vi "S-Curve2.vi"(8 "Conditions":T1, 9 "dt (s)":dbl=1.0, 10 "goal":dbl, 11 "Limits":T2) -> (0 "X":dbl[](array[numeric]), 1 "T":dbl[](array[numeric]), 3 "V":dbl[](array[numeric]))   [LabVIEW 2020]
uses:
  sub-vi/Sigmoid.vi
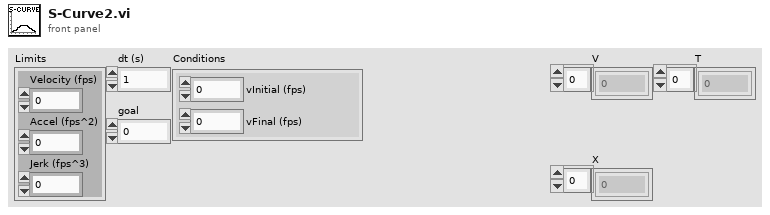
[diagram p1: front panel]
types:
  T1 = cluster{"vInitial (fps)":dbl, "vFinal (fps)":dbl}
  T2 = cluster{"Velocity (fps)":dbl, "Accel (fps^2)":dbl, "Jerk (fps^3)":dbl}
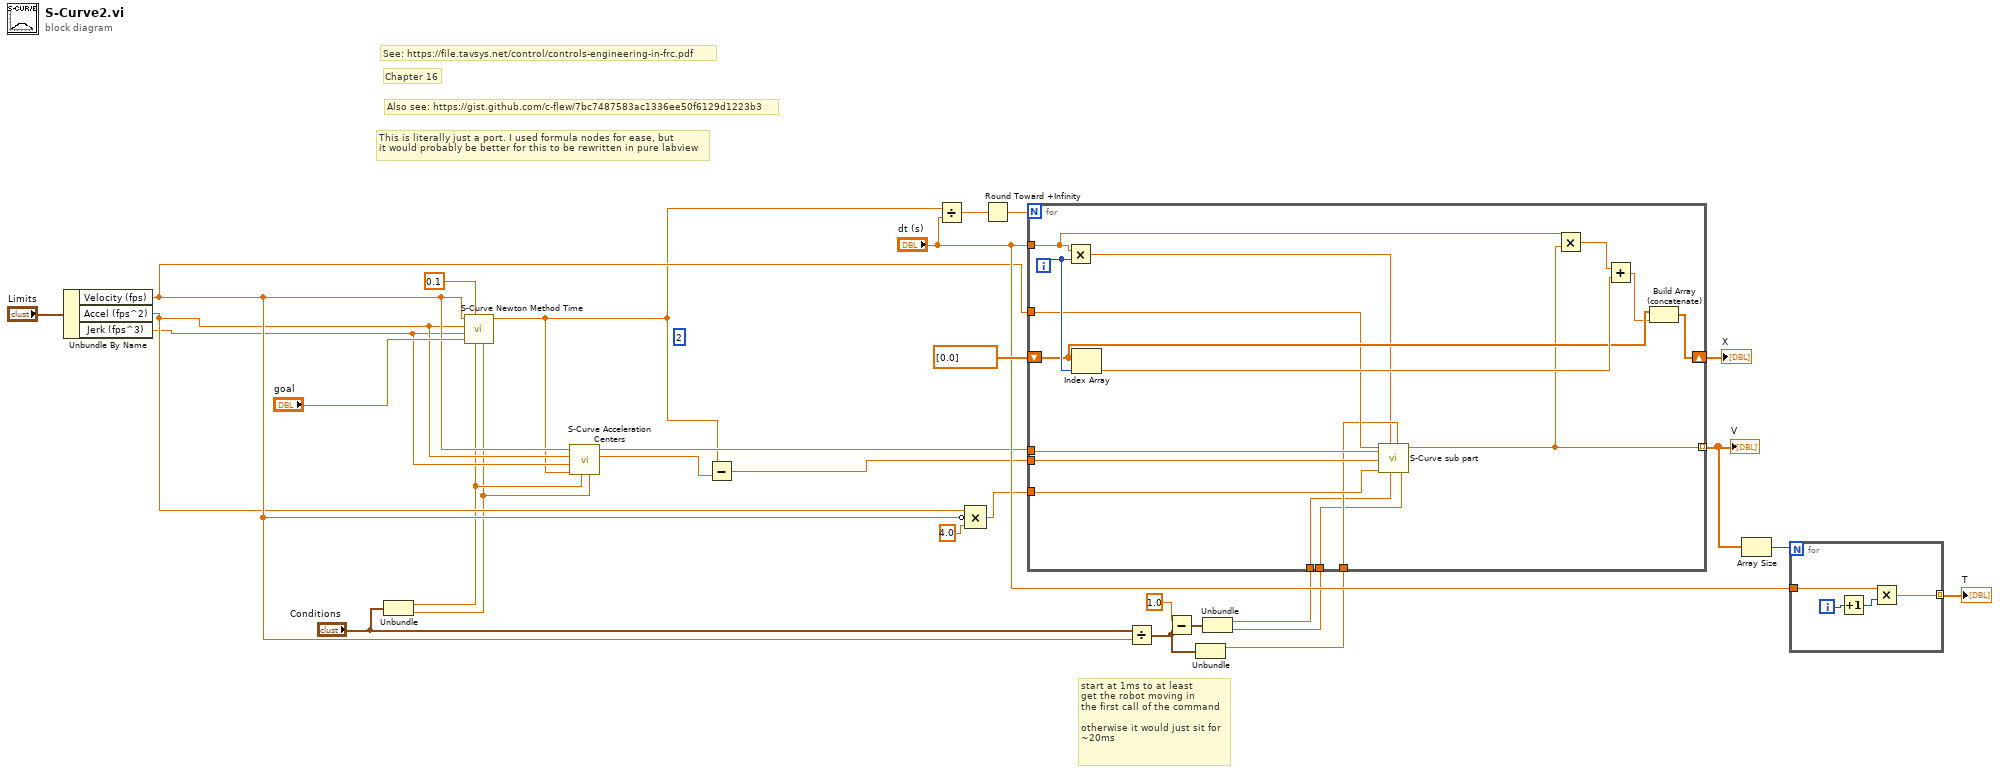
[diagram p0: block diagram]
diagram:
  (unwired) 2
  # "This is literally just a port. I used formula nodes for ease, but\nit would probably be better for this to be rewritten in pure labview"
  # "Also see: https://gist.github.com/c-flew/7bc7487583ac1336ee50f6129d1223b3"
  # "Chapter 16"
  # "See: https://file.tavsys.net/control/controls-engineering-in-frc.pdf"
  # "start at 1ms to at least\nget the robot moving in\nthe first call of the command\n\notherwise it would just sit for \n~20ms"
  n1 = Unbundle By Name("Limits") -> ("Velocity (fps)"=w8:dbl, "Accel (fps^2)"=w7:dbl, "Jerk (fps^3)"=w6:dbl)
  n2 = Unbundle("Conditions") -> ("vInitial (fps)"=w5:dbl, "vFinal (fps)"=w4:dbl)
  n3 = call "S-Curve Newton Method Time.vi"("v_f"=w4, "v_i"=w5, "err"=0.1, "g"="goal", "j"=w6, "a"=w7, "v"=w8) -> ("t_out"=w3:dbl)  [unwired: 4 in]
  n4 = call "S-Curve Acceleration Centers.vi"("v_f"=w4, "v_i"=w5, "t"=w3, "j"=w6, "a"=w7, "v"=w8) -> ("c2"=w2:dbl, "c1"=w9:dbl)  [unwired: 4 in]
  n5 = Subtract(x=w3, y=w2) -> (x-y=w1:dbl)
  n6 = Divide(x=w3, y="dt (s)") -> (x/y=w28:dbl)
  n7 = Compound Arithmetic op=MULTIPLY(w7, invert w8, 4.0 ("value")) -> (w14:dbl)
  n8 = Round Toward +Infinity(x=w28) -> (ceil(x): smallest int >= x=w27:dbl)
  n9 = Divide(x="Conditions", y=w8) -> (x/y=w20:T1)
  n10 = Subtract(x=1.0, y=w20) -> (x-y=w19:T1)
  n11 = Unbundle(w20) -> ("vInitial (fps)"=w16:dbl)  [unwired: 1 out]
  n12 = Unbundle(w19) -> ("vInitial (fps)"=w18:dbl, "vFinal (fps)"=w17:dbl)
  n13 = for {
    N: w27 -> [_]
    tunnel: "dt (s)" -> [w45]
    tunnel: w8 -> [w35]
    tunnel: w1 -> [w37]
    tunnel: w9 -> [w38]
    shift-right: [w39] -> w22
    shift-left: dbl[] [0.0] ("appended array") -> [w41]
    tunnel: w18 -> [w32]
    tunnel: w17 -> [w31]
    tunnel: w16 -> [w34]
    tunnel: w14 -> [w36]
    tunnel: [w30] -> w13 mode=indexing
    i -> [w44]
    n14 = Multiply(x=w45, y=w44) -> (x*y=w33:dbl)
    n15 = Index Array(array=w41, index=w44) -> (element=w42:dbl)
    n16 = call "S-Curve sub part.vi"("1-(v_f/v)"=w31, "v_i/v"=w34, "1-(v_i/v)"=w32, "x"=w33, "4a/v"=w36, "t-c2"=w37, "c1"=w38, "v"=w35) -> ("v_out"=w30:dbl)  [unwired: 3 in]
    n17 = Multiply(x=w45, y=w30) -> (x*y=w43:dbl)
    n18 = Add(x=w43, y=w42) -> (x+y=w40:dbl)
    n19 = Build Array (concatenate)(w41, w40) -> (w39:dbl[])
  }
  "V" <- w13
  "X" <- w22
  n20 = Array Size(array=w13) -> (size(s)=w25:i32)
  n21 = for {
    N: w25 -> [_]
    tunnel: "dt (s)" -> [w49]
    tunnel: [w48] -> w23 mode=indexing
    i -> [w47]
    n22 = Increment(x=w47) -> (x+1=w46:i32)
    n23 = Multiply(x=w49, y=w46) -> (x*y=w48:dbl)
  }
  "T" <- w23
